vi "factorial using shift register.vi"() -> ()   [LabVIEW 2018]
panel:
  out "Loop Count":i32
  out "result":u32
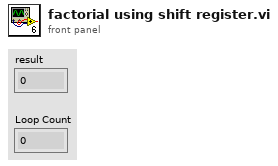
[diagram p1: front panel]
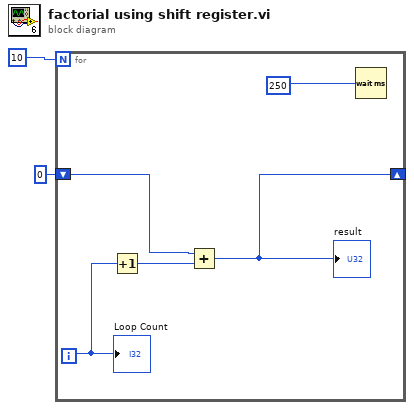
[diagram p0: block diagram]
diagram:
  n1 = for {
    N: 10 -> [_]
    shift-right: [w3] -> _
    shift-left: 0 -> [w4]
    i -> [w6]
    n2 = Increment(x=w6) -> (x+1=w5:i32)
    n3 = Add(x=w4, y=w5) -> (x+y=w3:i32)
    "result" <- w3
    n4 = Wait (ms)(milliseconds to wait=u32 250) -> ()  [unwired: 1 out]
    "Loop Count" <- w6
  }
